vi "lv-ros-bridge_READ copy.vi"(8 "error in (no error)":errorcluster, 9 "Topic to subscribe":string="/", 10 "rosbridge port":u16=9090, 11 "rosbridge server IP":string="192.168.164.128") -> (0 "error out":errorcluster)   [LabVIEW 2015]
uses:
  <vilib>/MediaMongrels Ltd/WebSockets/WebSockets/WebSockets.lvlib
panel:
  out "Return Headers Out":variant
  in  "error in (no error) 3":errorcluster
  in  "rosbridge port 3":u16=9090
  in  "rosbridge server IP 3":string="192.168.1.117"
  out "Data 2":string
  out "Opcode 2":u8
  in  "szablon 2":T1
  in  "stop 2":bool
  out "value 3":T1
  out "error out 2":errorcluster
  in  "Topic to subscribe 2":string="/"
  out "value 2":T2
  in  "STEERING":T2
  out "value":T1
  in  "szablon":T1
  out "Opcode":u8
  out "Data":string
  in  "stop":bool
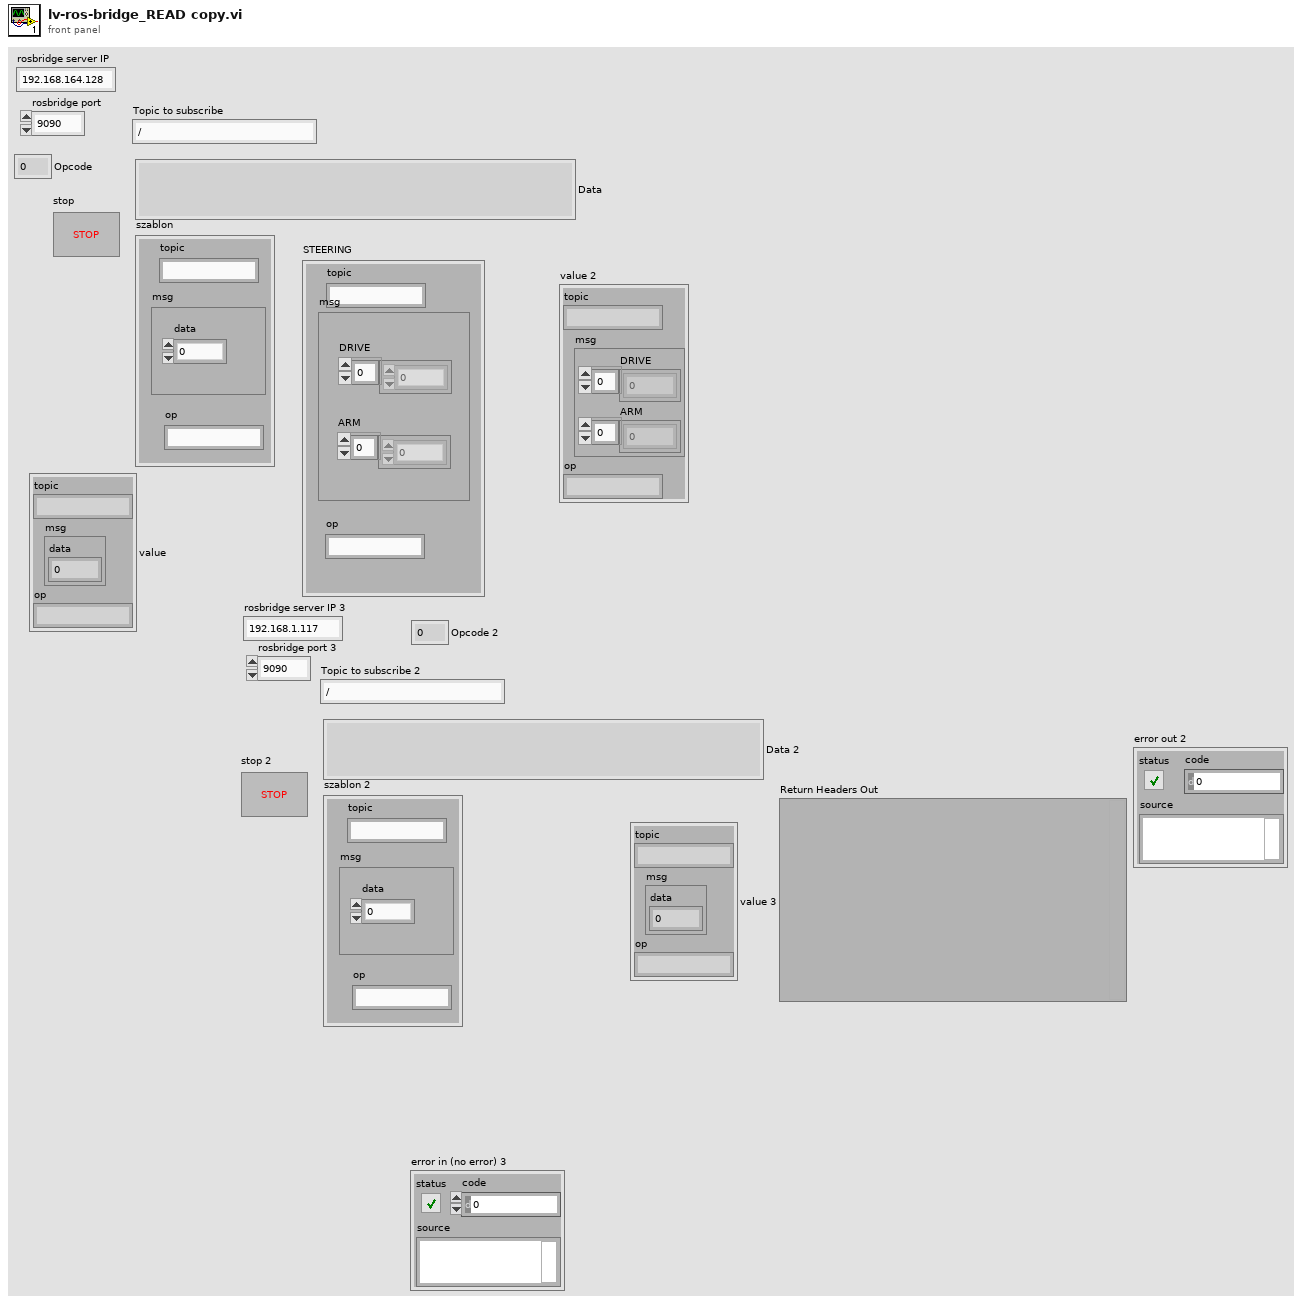
[diagram p1: front panel]
types:
  T1 = cluster{"topic":string, "msg":cluster{"data":i16}, "op":string}
  T2 = cluster{"topic":string, "msg":cluster{"DRIVE":i16[], "ARM":i8[]}, "op":string}
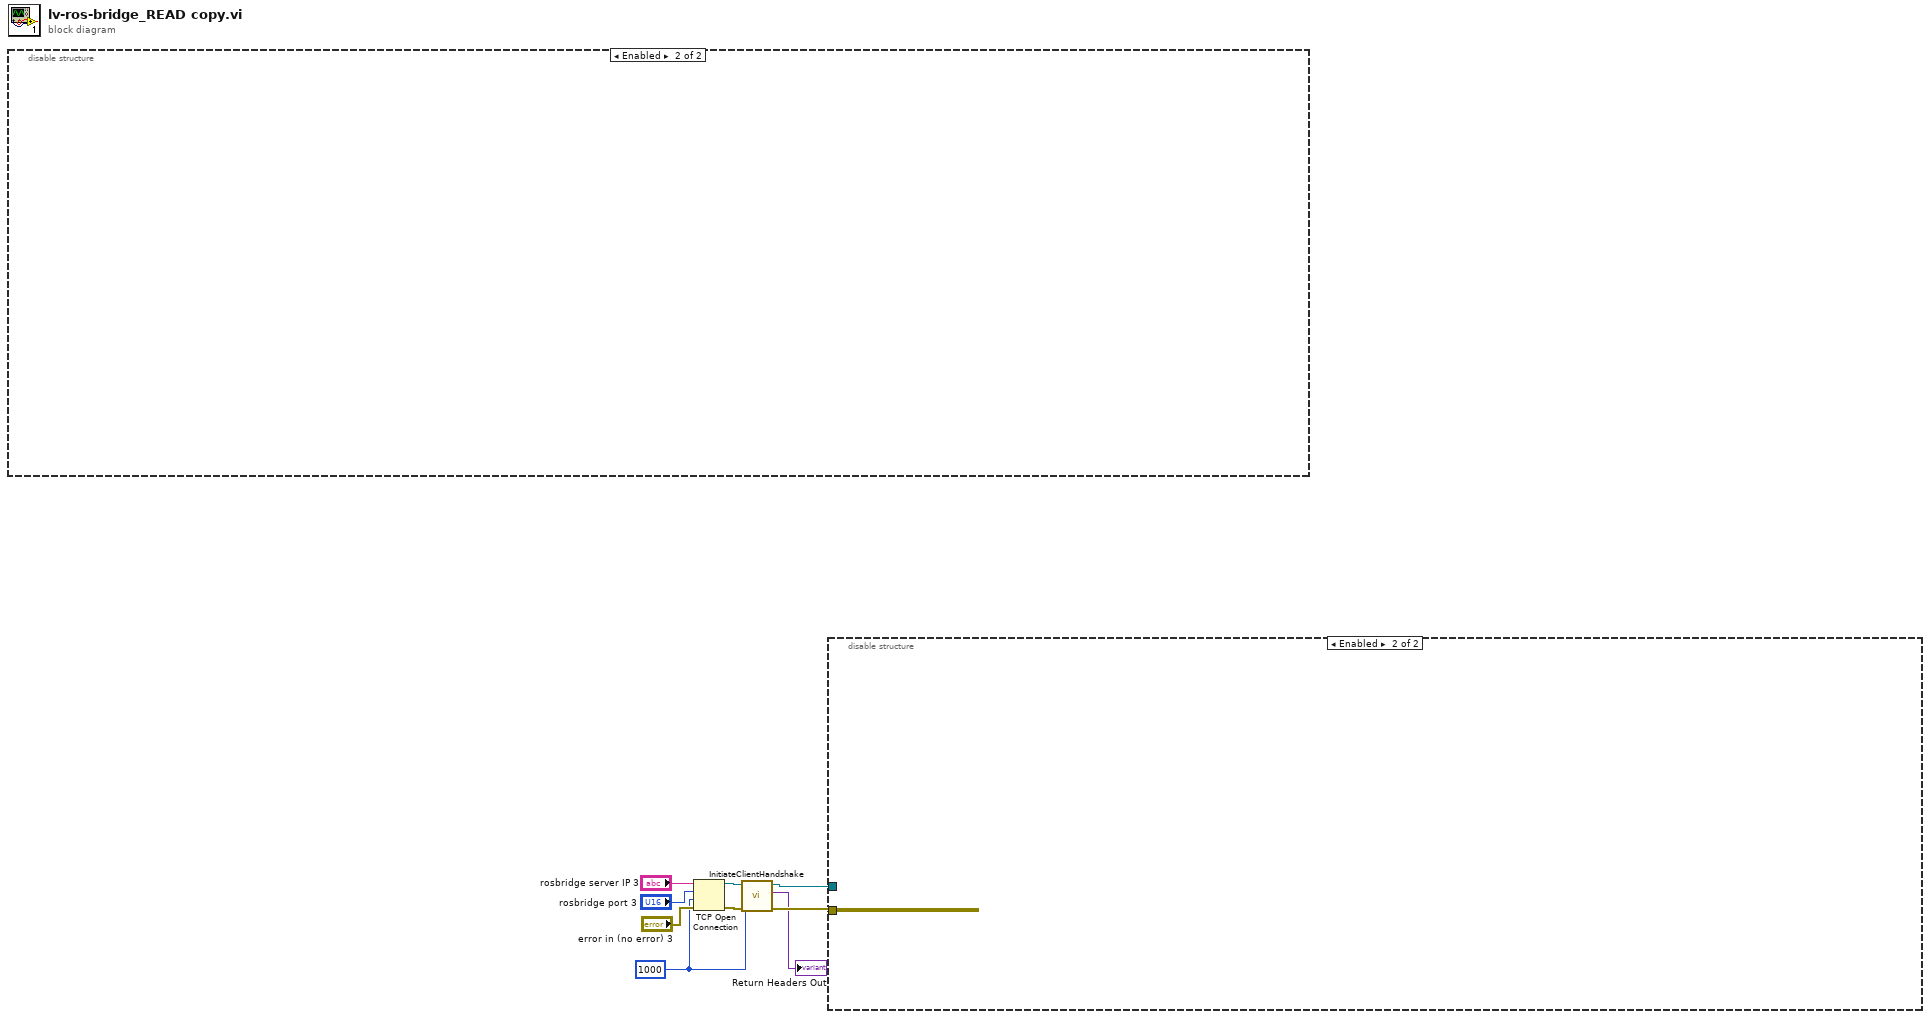
[diagram p0: block diagram]
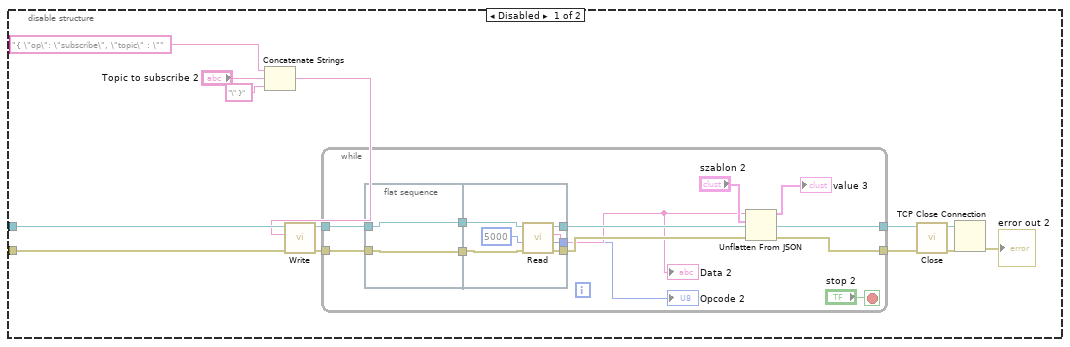
[diagram p2: hidden frame]
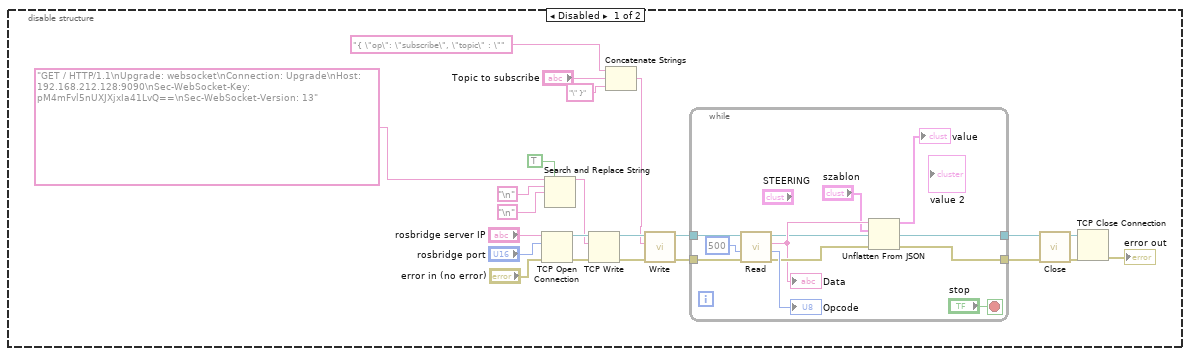
[diagram p3: hidden frame]
diagram:
  w1 = 1000 ("timeout ms (5000)")
  n1 = disable-structure shown="Enabled" {
    frame Disabled {
      n2 = TCP Open Connection(address="rosbridge server IP", remote port or service name="rosbridge port", error in (no error)="error in (no error)") -> (connection ID=w30:refnum<k5>, error out=w29:errorcluster)  [unwired: 2 in]
      n3 = Search and Replace String(replace all?=TRUE ("replace all? (F)"), input string="GET / HTTP/1.1\nUpgrade: websocket\nConnection: Upgrade\nHost: 192.168.212.128:9090\nSec-WebSocket-Key: pM4mFvl5nUXJXjxIa41LvQ==\nSec-WebSocket-Version: 13", search string="\n", replace string="\n") -> (result string=w15:string)  [unwired: 4 in, 3 out]
      n4 = TCP Write(connection ID=w30, data in=w15, error in (no error)=w29) -> (connection ID out=w26:refnum<k5>, error out=w25:errorcluster)  [unwired: 1 in, 1 out]
      n5 = Concatenate Strings("{ \"op\": \"subscribe\", \"topic\" : \"", "Topic to subscribe", "\" }") -> (w13:string)
      n6 = call <vilib>:"Write.vi"("error in (no error)"=w25, "Data"=w13, "WebSocket Connection in"=w26) -> ("error out"=w21:errorcluster, "WebSocket Connection out"=w22:refnum<k5>)  [unwired: 7 in]
      n7 = while {
        tunnel: [w36] -> w24
        tunnel: [w35] -> w23
        tunnel: w22 -> [w43]
        tunnel: w21 -> [w42]
        stop <- "stop" stop-if-true
        n8 = call <vilib>:"Read.vi"("error in (no error)"=w42, "timeout ms (5000)"=500, "WebSocket Connection in"=w43) -> ("error out"=w39:errorcluster, "Opcode"=→"Opcode":u8, "Data"=w38:string, "WebSocket Connection out"=w36:refnum<k5>)  [unwired: 5 in]
        "Data" <- w38
        n9 = Unflatten From JSON(JSON string=w38, type and defaults="szablon", error in (no error)=w39) -> (value=→"value":T1, error out=w35:errorcluster)  [unwired: 4 in]
      }
      n10 = call <vilib>:"Close.vi"("error in (no error)"=w23, "WebSocket Connection in"=w24) -> ("error out"=w27:errorcluster, "WebSocket Connection in"=w28:refnum<k5>)  [unwired: 8 in]
      n11 = TCP Close Connection(connection ID=w28, error in (no error)=w27) -> (error out=→"error out":errorcluster)  [unwired: 1 in, 1 out]
    }
    frame Enabled {
    }
  }
  n12 = TCP Open Connection(address="rosbridge server IP 3", remote port or service name="rosbridge port 3", timeout ms (60000)=w1, error in (no error)="error in (no error) 3") -> (connection ID=w6:refnum<k5>, error out=w7:errorcluster)  [unwired: 1 in]
  n13 = call <vilib>:"InitiateClientHandshake.vi"("error in (no error)"=w7, "timeout ms (5000)"=w1, "WebSocket Connection in"=w6) -> ("error out"=w8:errorcluster, "Return Headers Out"=→"Return Headers Out":variant, "WebSocket Connection out"=w9:refnum<k5>)  [unwired: 6 in]
  n14 = disable-structure shown="Enabled" {
    disable-tunnel: w9 -> [w54 _]
    disable-tunnel: w8 -> [w53 _]
    frame Disabled {
      n15 = Concatenate Strings("{ \"op\": \"subscribe\", \"topic\" : \"", "Topic to subscribe 2", "\" }") -> (w46:string)
      n16 = call <vilib>:"Write.vi"("error in (no error)"=w53, "Data"=w46, "WebSocket Connection in"=w54) -> ("error out"=w49:errorcluster, "WebSocket Connection out"=w50:refnum<k5>)  [unwired: 7 in]
      n17 = while {
        tunnel: [w60] -> w52
        tunnel: [w65] -> w51
        tunnel: w50 -> [w64]
        tunnel: w49 -> [w63]
        stop <- "stop 2" stop-if-true
        n18 = flat-sequence {
          tunnel: w64 -> [w69]
          tunnel: w63 -> [w70]
          tunnel: [w70] -> w62
          tunnel: [w69] -> w61
          tunnel: w62 -> [w75]
          tunnel: w61 -> [w76]
          tunnel: [w74] -> w60
          tunnel: [w73] -> w59
          tunnel: [w72] -> w58
          tunnel: [w71] -> w57
          frame #0 {
          }
          frame #1 {
            n19 = call <vilib>:"Read.vi"("error in (no error)"=w75, "timeout ms (5000)"=5000, "WebSocket Connection in"=w76) -> ("error out"=w73:errorcluster, "Opcode"=w71:u8, "Data"=w72:string, "WebSocket Connection out"=w74:refnum<k5>)  [unwired: 5 in]
          }
        }
        n20 = Unflatten From JSON(JSON string=w58, type and defaults="szablon 2", error in (no error)=w59) -> (value=→"value 3":T1, error out=w65:errorcluster)  [unwired: 4 in]
        "Data 2" <- w58
        "Opcode 2" <- w57
      }
      n21 = call <vilib>:"Close.vi"("error in (no error)"=w51, "WebSocket Connection in"=w52) -> ("error out"=w55:errorcluster, "WebSocket Connection in"=w56:refnum<k5>)  [unwired: 8 in]
      n22 = TCP Close Connection(connection ID=w56, error in (no error)=w55) -> (error out=→"error out 2":errorcluster)  [unwired: 1 in, 1 out]
    }
    frame Enabled {
    }
  }
